vi "serial_read_write.vi"() -> ()   [LabVIEW 2018]
uses:
  <vilib>/Instr/_visa.llb/VISA Configure Serial Port (Instr).vi
panel:
  out "return count":u32
  out "read buffer":string
  in  "stop bits (10: 1 bit)":u16(ring)=10 items=["1.0"=10, "1.5"=15, "2.0"=20]
  in  "parity (0:none)":enum16{"None", "Odd", "Even", "Mark", "Space"}(ring)
  in  "data bits (8)":u16=8 min=5 max=8 step=1
  in  "baud rate (9600)":u32=9600
  in  "VISA resource name":refnum<visa-resource-name>
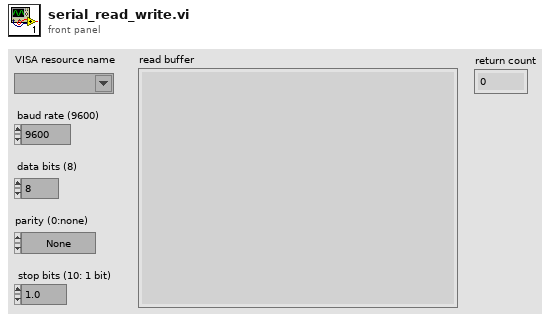
[diagram p1: front panel]
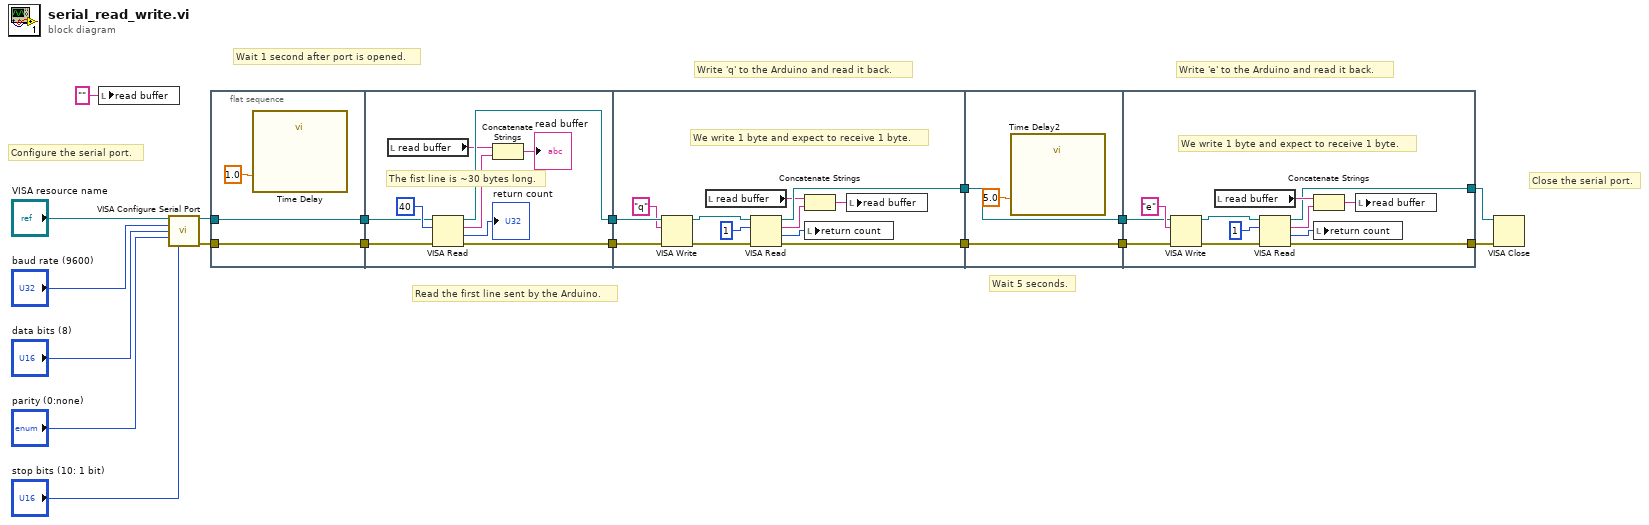
[diagram p0: block diagram]
diagram:
  # "Close the serial port."
  # "Configure the serial port."
  # "Write 'e' to the Arduino and read it back."
  # "Wait 5 seconds."
  # "Write 'q' to the Arduino and read it back."
  # "Read the first line sent by the Arduino."
  # "Wait 1 second after port is opened."
  n1 = local write "read buffer"("" ("read buffer")) -> ()
  n2 = call-poly "VISA Configure Serial Port"("VISA resource name"="VISA resource name", "baud rate (9600)"="baud rate (9600)", "data bits (8)"="data bits (8)", "parity (0:none)"="parity (0:none)", "stop bits (10: 1 bit)"="stop bits (10: 1 bit)") -> ("VISA resource name out"=w13:refnum<visa-resource-name>, "error out"=w12:errorcluster)  [unwired: 9 in]
  n3 = flat-sequence {
    tunnel: w12 -> [w20]
    tunnel: w13 -> [w21]
    tunnel: [w21] -> w3
    tunnel: [w20] -> w2
    tunnel: [w30] -> w11
    tunnel: [w28] -> w9
    tunnel: w3 -> [w22]
    tunnel: w2 -> [w29]
    tunnel: w11 -> [w42]
    tunnel: [w40] -> w10
    tunnel: w9 -> [w39]
    tunnel: [w37] -> w8
    tunnel: w10 -> [w45]
    tunnel: w8 -> [w44]
    tunnel: [w45] -> w7
    tunnel: [w44] -> w6
    tunnel: w7 -> [w49]
    tunnel: w6 -> [w48]
    tunnel: [w47] -> w5
    tunnel: [w46] -> w4
    frame #0 {
      n4 = call "Time Delay"("Delay Time (s)"=1.0) -> ()  [unwired: 10 in, 1 out]
    }
    frame #1 {
      # "The fist line is ~30 bytes long."
      n5 = local read "read buffer"() -> (w24:string)
      n6 = VISA Read(VISA resource name=w22, byte count=u32 40, error in (no error)=w29) -> (VISA resource name out=w30:refnum<visa-resource-name>, read buffer=w25:string, return count=→"return count":u32, error out=w28:errorcluster)
      n7 = Concatenate Strings(w24, w25) -> (→"read buffer":string)
    }
    frame #2 {
      # "We write 1 byte and expect to receive 1 byte."
      n8 = VISA Write(VISA resource name=w42, write buffer="q", error in (no error)=w39) -> (VISA resource name out=w41:refnum<visa-resource-name>, error out=w38:errorcluster)  [unwired: 1 out]
      n9 = local read "read buffer"() -> (w31:string)
      n10 = VISA Read(VISA resource name=w41, byte count=u32 1, error in (no error)=w38) -> (VISA resource name out=w40:refnum<visa-resource-name>, read buffer=w32:string, return count=w34:u32, error out=w37:errorcluster)
      n11 = Concatenate Strings(w31, w32) -> (w33:string)
      n12 = local write "return count"(w34) -> ()
      n13 = local write "read buffer"(w33) -> ()
    }
    frame #3 {
      n14 = call "Time Delay2"("Delay Time (s)"=5.0) -> ()  [unwired: 10 in, 1 out]
    }
    frame #4 {
      # "We write 1 byte and expect to receive 1 byte."
      n15 = VISA Write(VISA resource name=w49, write buffer="e", error in (no error)=w48) -> (VISA resource name out=w57:refnum<visa-resource-name>, error out=w56:errorcluster)  [unwired: 1 out]
      n16 = local read "read buffer"() -> (w50:string)
      n17 = VISA Read(VISA resource name=w57, byte count=u32 1, error in (no error)=w56) -> (VISA resource name out=w47:refnum<visa-resource-name>, read buffer=w51:string, return count=w53:u32, error out=w46:errorcluster)
      n18 = Concatenate Strings(w50, w51) -> (w52:string)
      n19 = local write "return count"(w53) -> ()
      n20 = local write "read buffer"(w52) -> ()
    }
  }
  n21 = VISA Close(VISA resource name=w5, error in (no error)=w4) -> ()  [unwired: 1 out]
